vi "ALTS-2015 Test Type Selection.vi"(8 "error in (no error)":errorcluster, 9 "Timeout (10000ms)":i32=10000, 11 "Station Cluster":T1) -> (0 "error out":errorcluster, 3 "Test Type Selection Successful":bool)   [LabVIEW 2013]
uses:
  Controls/ALTS-2015 Station Cluster.ctl
  Controls/ALTS-2015 LV2GBL Station Info Options.ctl
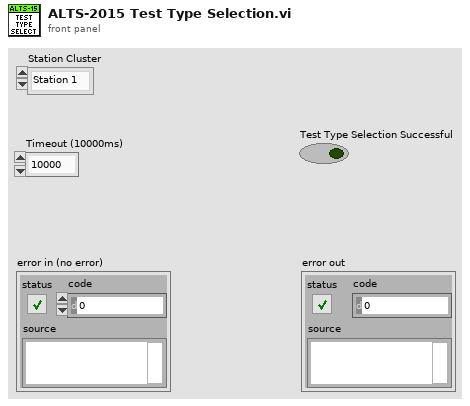
[diagram p1: front panel]
types:
  T1 = typedef "ALTS-2015 Station Cluster.ctl" = enum16{"Station 1", "Station 2", "Station 3", "Station 4"}
  T2 = typedef "ALTS-2015 LV2GBL Station Info Options.ctl" = enum16{"Init", "Read", "Read All", "Write Sensor ID", "Write  Work Order", "Write Serial Number", "Write Test Data", "Write Station Status", "Write Station Occupancy", "Write Station Test Type", "Write Rerun", "Write Load Decision", "Clear All", "Clear Test Result"}
  T3 = typedef "ALTS-2015 Station Details.ctl" = cluster{"Station Number":string, "Work Order Number":string, "Sensor Name":string, "Pressure (PSI)":string, "Flow (SCCM)":string, "Test Time ":string, "Test Result":string, "Serial Number":string, "Station Status":T4, "Station Occupied?":bool, "Rerun Count":i32, "Test Type":i32}
  T4 = typedef "ALTS-2015 Status Ring Indicator.ctl" = u16
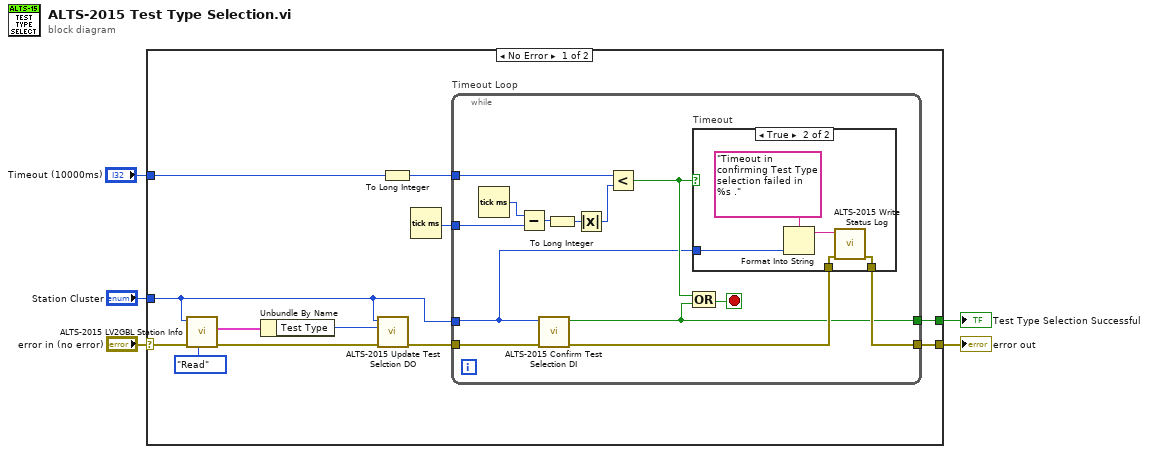
[diagram p0: block diagram]
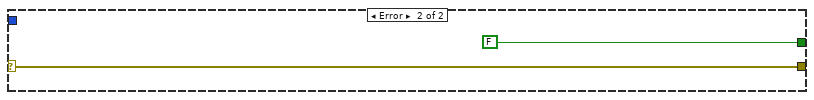
[diagram p3: hidden frame]
diagram:
  n1 = case shown="No Error" "error in (no error)" {
    selector: "error in (no error)" -> [w10 w38]
    tunnel: "Station Cluster" -> [w15 _]
    tunnel: [w12 FALSE ("Test Type Selection Successful")] -> w4
    tunnel: [w11 w38] -> w3
    tunnel: "Timeout (10000ms)" -> [w7 _]
    frame No Error {
      n2 = call "ALTS-2015 LV2GBL Station Info.vi"("Options"=ALTS-2015_LV2GBL_Station_Info_Options."Read", "error in"=w10, "Station Cluster"=w15) -> ("error out"=w14:errorcluster, "Station Details"=w16:T3)  [unwired: 4 in, 3 out]
      n3 = Unbundle By Name(w16) -> ("Test Type"=w17:i32)
      n4 = call "ALTS-2015 Update Test Selction DO.vi"("error in"=w14, "Test Type In"=w17, "Station Cluster"=w15) -> ("error out"=w13:errorcluster)  [unwired: 8 in]
      n5 = To Long Integer(number=w7) -> (32bit integer=w8:i32)
      n6 = Tick Count (ms)() -> (millisecond timer value=w9:u32)
      n7 = while "Timeout Loop" {
        tunnel: w15 -> [w18]
        tunnel: w13 -> [w30]
        tunnel: [w19] -> w12
        tunnel: [w22] -> w11
        tunnel: w9 -> [w25]
        tunnel: w8 -> [w24]
        stop <- w23 stop-if-true
        n8 = Tick Count (ms)() -> (millisecond timer value=w26:u32)
        n9 = Subtract(x=w26, y=w25) -> (x-y=w28:u32)
        n10 = call "ALTS-2015 Confirm Test Selection DI.vi"("error in"=w30, "Station Cluster"=w18) -> ("error out"=w20:errorcluster, "Test Type Selection Successful"=w19:bool)  [unwired: 8 in]
        n11 = To Long Integer(number=w28) -> (32bit integer=w27:i32)
        n12 = Absolute Value(x=w27) -> (abs(x)=w29:i32)
        n13 = Less?(x=w24, y=w29) -> (x < y?=w21:bool)
        n14 = case "Timeout" shown="True" w21 {
          tunnel: w20 -> [w31 w36]
          tunnel: [w31 w35] -> w22
          tunnel: w18 -> [_ w32]
          frame False {
            # "Test Type Selection is successful"
          }
          frame True {
            n15 = Format Into String(format string="Timeout in confirming Test Type selection failed in %s ." ("Status Input"), w32) -> (resulting string=w33:string)  [unwired: 2 in, 1 out]
            n16 = call "ALTS-2015 Write Status Log.vi"("error in (no error)"=w36, "Status Input"=w33) -> ("error out"=w35:errorcluster)  [unwired: 9 in]
          }
        }
        n17 = Compound Arithmetic op=OR(w21, w19) -> (w23:bool)
      }
    }
    frame Error {
    }
  }
  "Test Type Selection Successful" <- w4
  "error out" <- w3
